vi "main 3rd.vi"() -> ()   [LabVIEW 2013]
uses:
  <vilib>/Utility/file.llb/Read From Spreadsheet File (DBL).vi
panel:
  out "数值 2":i32
  out "数值":i32
  out "From OD fit?":bool
  out "Current file num":i32
  out "ROI Width":u32
  out "ROI Height":u32
  in  "Image Dark":dbl[][](array[numeric])
  in  "Image Light":dbl[][](array[numeric])
  in  "Image Atom":dbl[][](array[numeric])
  out "Best fit parameters":dbl[](array[numeric])
  out "Fitting Results Save Path":string[](array[string])
  out "Best fit results":dbl[][](array[numeric])
  in  "Initial guess values":dbl[](array[numeric])
  in  "Latest image data":dbl[][](array[numeric])
  out "Fitting Type":u16(ring)
  out "Force Guess?":bool
  out "Aquired?":bool
  out "Process Index":i32
  out "External Trigger":bool
  out "XY图":cluster{dbl[], dbl[]}[](graph)
  out "OD Image":dbl[][](graph)
  in  "OD fit":bool
  in  "OD num":i32
  out "Fit Done":bool
  in  "Exit":bool
  out "XY图 2":cluster{dbl[], dbl[]}[](graph)
  in  "Auto Split":bool
  in  "Fit":bool
  in  "Open File":bool
  in  "Auto Fit":bool
  in  "Stop":bool
  in  "Aquire":bool
  in  "Fitting Config":bool
  in  "Camera Config":bool
  in  "Initialize":bool
  in  "Live Image Display":refnum<k7>(container)
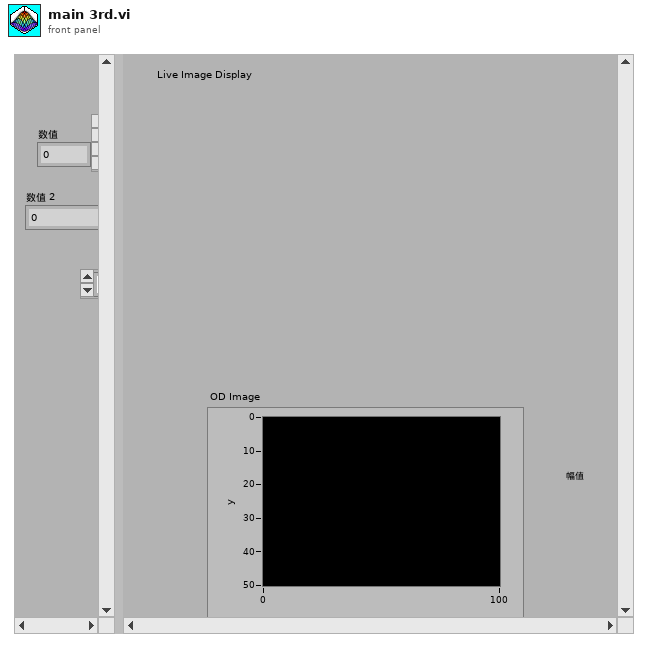
[diagram p1: front panel]
types:
  T1 = enum8{"Enabled", "Disabled", "Disabled and Grayed Out"}
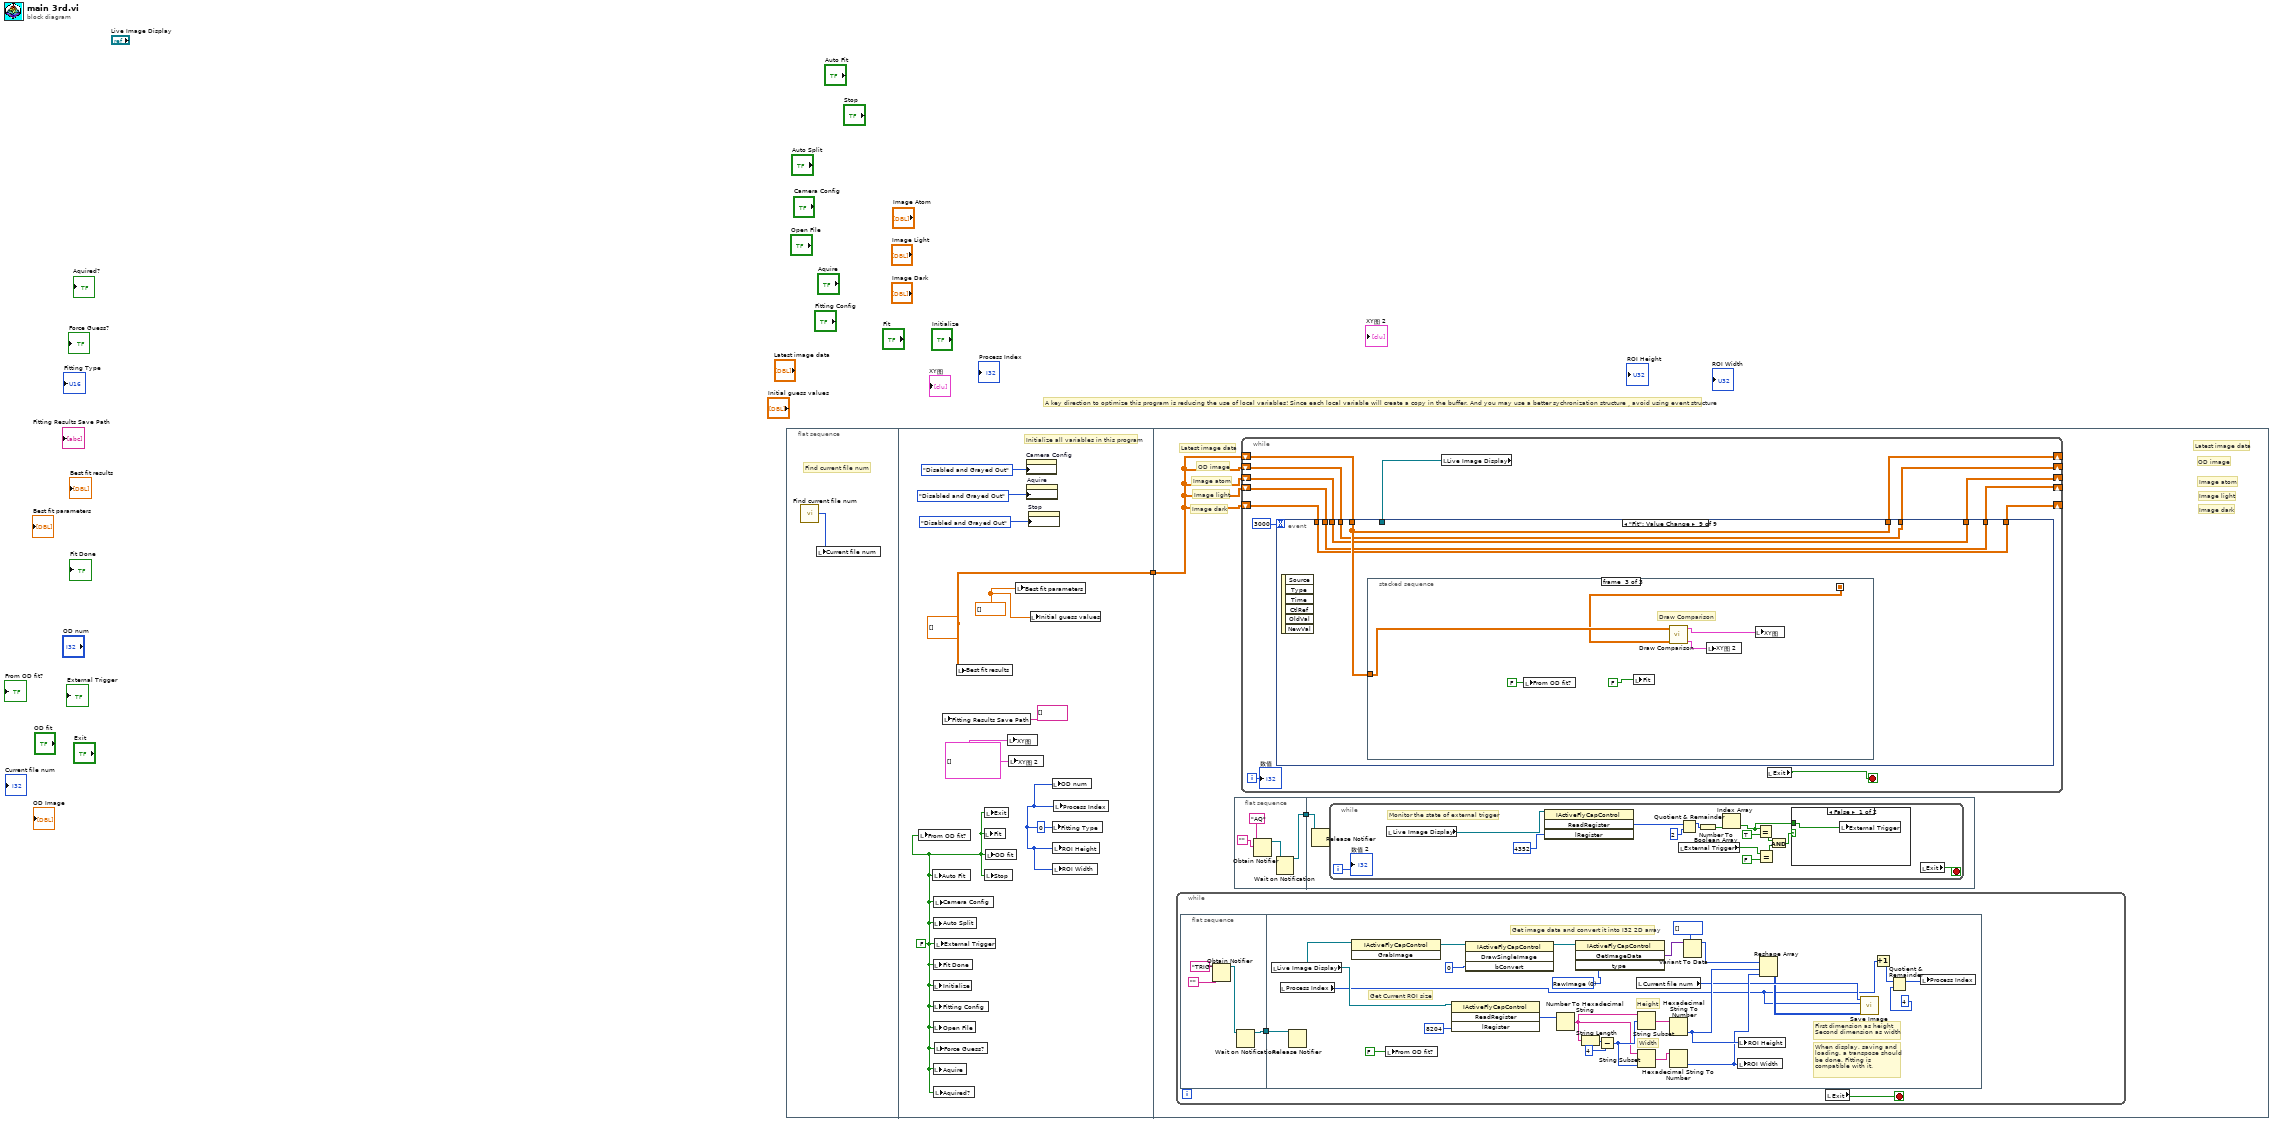
[diagram p0: block diagram]
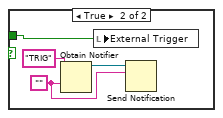
[diagram p2: hidden frame]
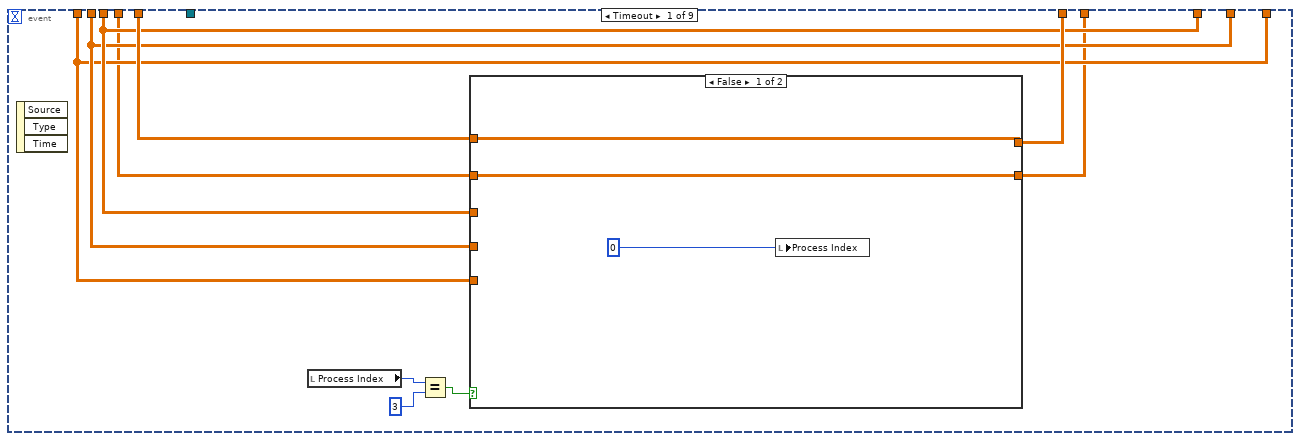
[diagram p3: hidden frame]
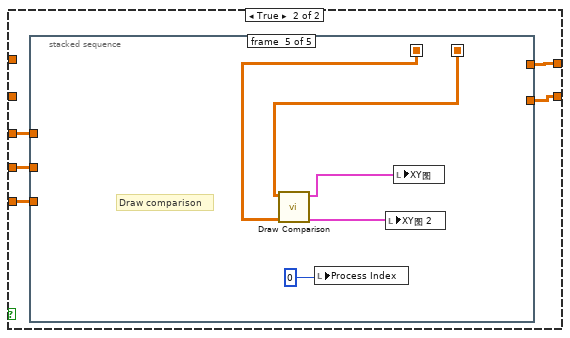
[diagram p4: hidden frame]
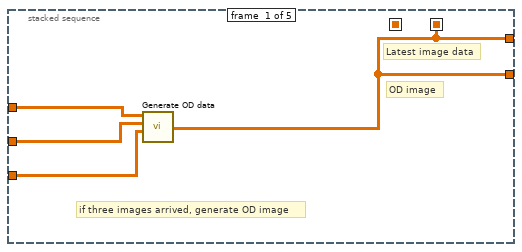
[diagram p5: hidden frame]
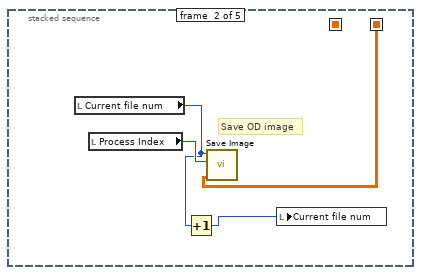
[diagram p6: hidden frame]
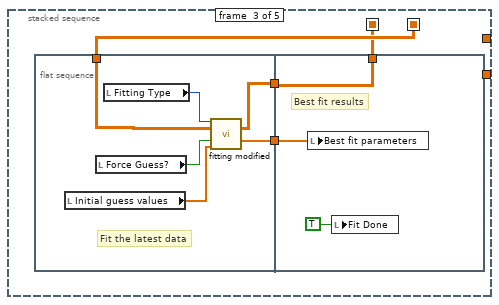
[diagram p7: hidden frame]
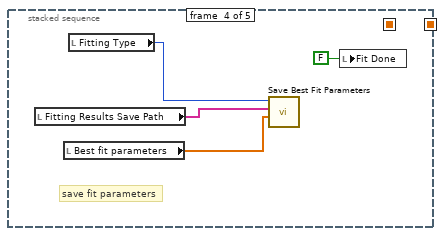
[diagram p8: hidden frame]
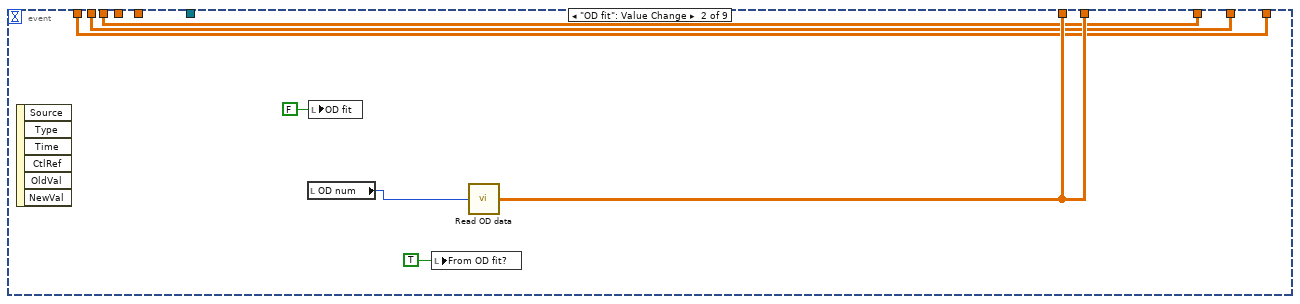
[diagram p9: hidden frame]
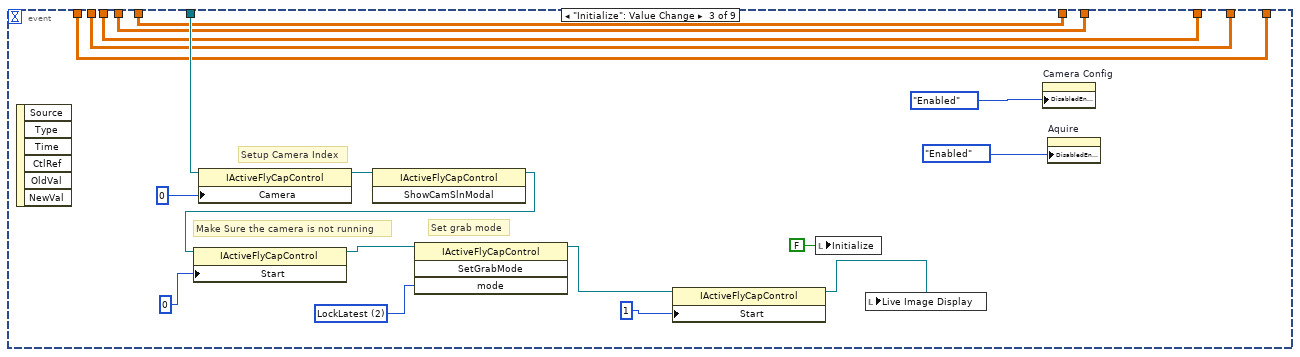
[diagram p10: hidden frame]
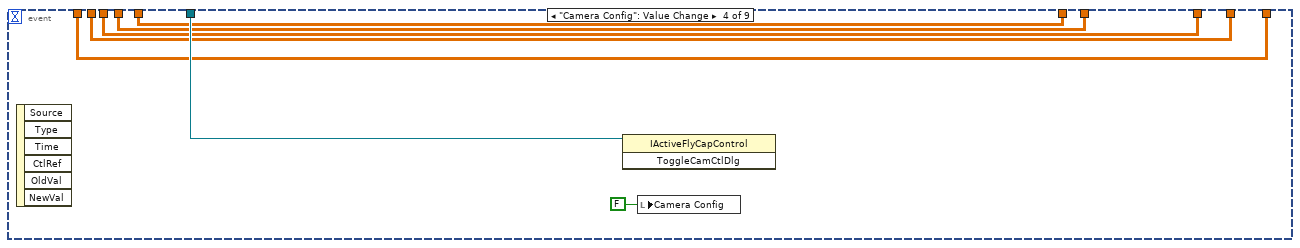
[diagram p11: hidden frame]
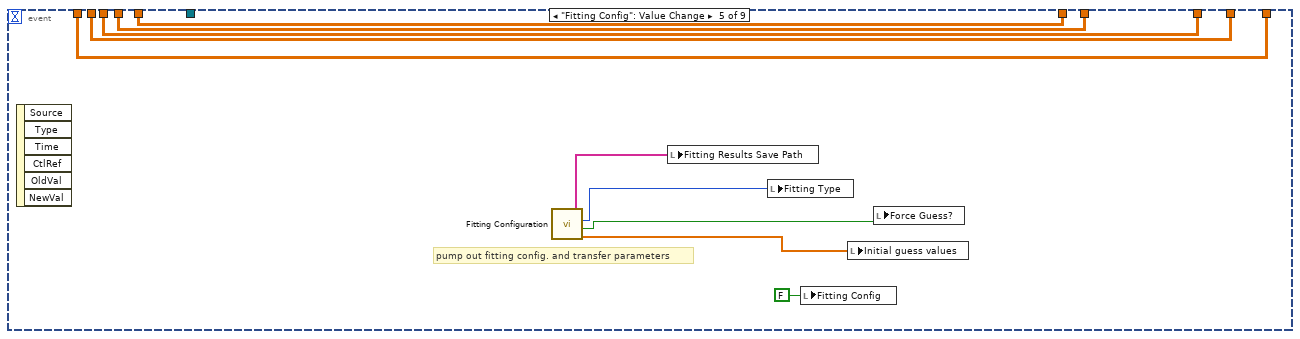
[diagram p12: hidden frame]
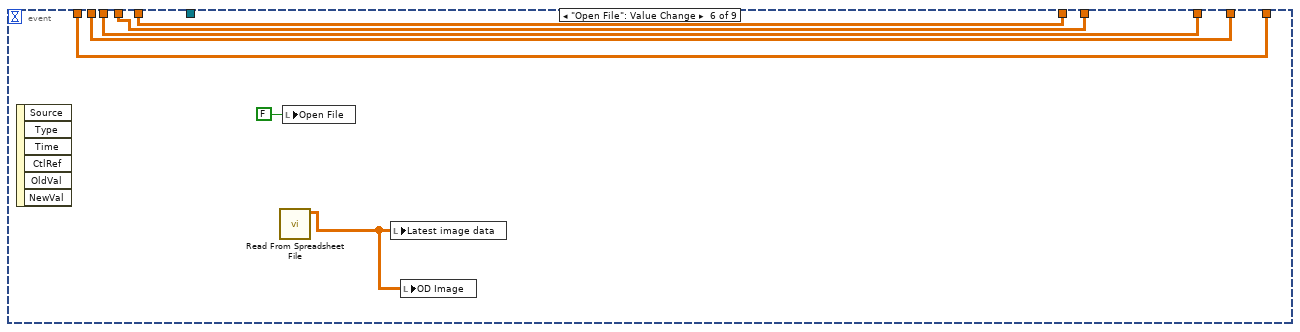
[diagram p13: hidden frame]
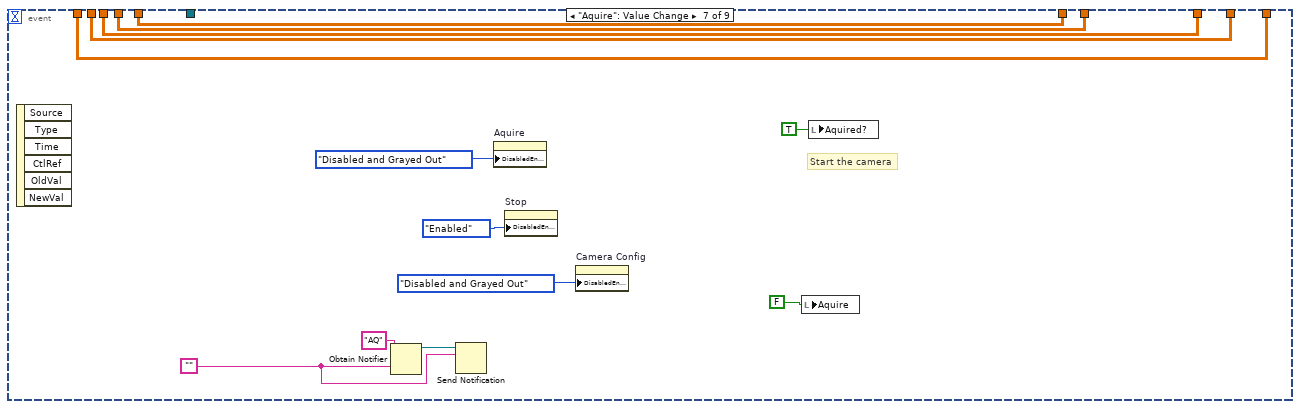
[diagram p14: hidden frame]
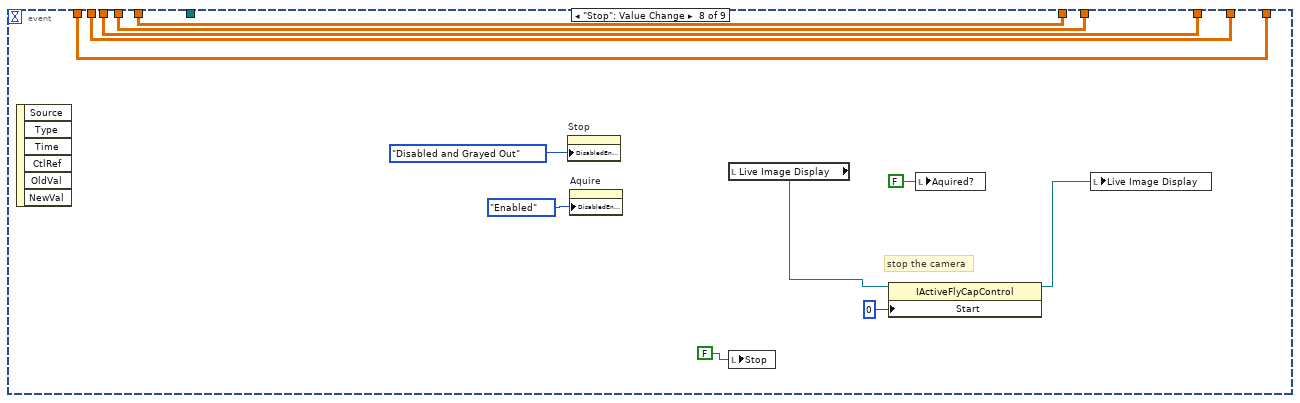
[diagram p15: hidden frame]
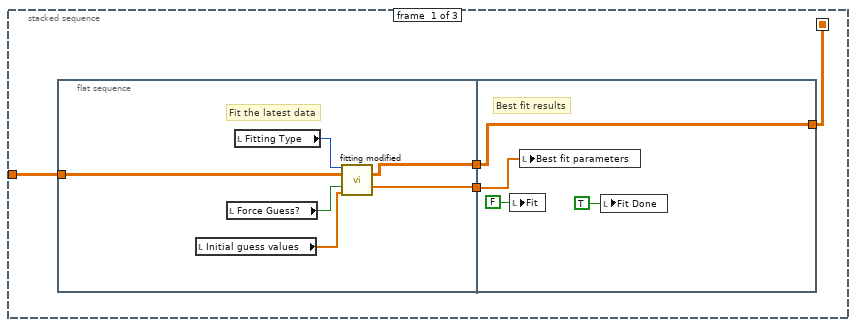
[diagram p16: hidden frame]
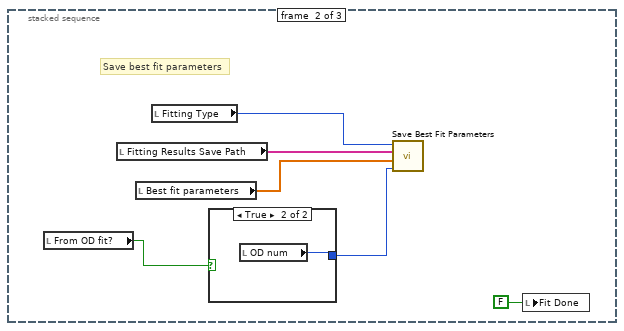
[diagram p17: hidden frame]
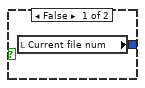
[diagram p18: hidden frame]
diagram:
  # "A key direction to optimize this program is reducing the use of local variables! Since each local variable will create a copy in the buffer. And you may use a better sychronization structure，avoid using event structure"
  n1 = flat-sequence {
    tunnel: [w5] -> w1
    tunnel: w1 -> [w13]
    frame #0 {
      # "Find current file num"
      n2 = call "Find current file num.vi"() -> ("Current File Num"=w2:u16)  [unwired: 2 in]
      n3 = local write "Current file num"(w2) -> ()
    }
    frame #1 {
      w7 = cluster{dbl[], dbl[]}[] [] ("XY图")
      w6 = 0 ("OD num")
      w5 = dbl[][] [] ("Best fit results")
      w4 = dbl[] [] ("Best fit parameters")
      w3 = FALSE ("Aquire")
      # "Initialize all variables in this program"
      n4 = local write "From OD fit?"(w3) -> ()
      n5 = local write "Auto Fit"(w3) -> ()
      n6 = local write "Auto Split"(w3) -> ()
      n7 = local write "Fit Done"(w3) -> ()
      n8 = local write "Initialize"(w3) -> ()
      n9 = local write "Fitting Config"(w3) -> ()
      n10 = local write "Open File"(w3) -> ()
      n11 = local write "Aquire"(w3) -> ()
      n12 = local write "Camera Config"(w3) -> ()
      n13 = local write "Aquired?"(w3) -> ()
      n14 = local write "Force Guess?"(w3) -> ()
      n15 = local write "External Trigger"(w3) -> ()
      n16 = local write "Fitting Results Save Path"(string[] [] ("Fitting Results Save Path")) -> ()
      n17 = local write "Best fit results"(w5) -> ()
      n18 = local write "Fit"(w3) -> ()
      n19 = local write "Exit"(w3) -> ()
      n20 = local write "Stop"(w3) -> ()
      n21 = local write "OD fit"(w3) -> ()
      n22 = local write "XY图"(w7) -> ()
      n23 = local write "XY图 2"(w7) -> ()
      n24 = local write "Best fit parameters"(w4) -> ()
      n25 = property on="Camera Config" class="Bool (strict)"("DisabledEnum"=T1."Disabled and Grayed Out" ("禁用")) -> ()  [unwired: 2 in, 2 out]
      n26 = property on="Aquire" class="Bool (strict)"("DisabledEnum"=T1."Disabled and Grayed Out" ("禁用")) -> ()  [unwired: 2 in, 2 out]
      n27 = property on="Stop" class="Bool (strict)"("DisabledEnum"=T1."Disabled and Grayed Out" ("禁用")) -> ()  [unwired: 2 in, 2 out]
      n28 = local write "Initial guess values"(w4) -> ()
      n29 = local write "OD num"(w6) -> ()
      n30 = local write "Fitting Type"(w6) -> ()
      n31 = local write "ROI Height"(w6) -> ()
      n32 = local write "ROI Width"(w6) -> ()
      n33 = local write "Process Index"(w6) -> ()
    }
    frame #2 {
      # "Image dark"
      # "Image light"
      # "Image atom"
      # "Image dark"
      # "Image light"
      # "Image atom"
      # "OD image"
      # "Latest image data"
      # "OD image"
      # "Latest image data"
      n34 = while {
        stop <- w40 stop-if-true
        n35 = flat-sequence {
          tunnel: [w41] -> w39
          tunnel: w39 -> [w53]
          frame #0 {
            n36 = Obtain Notifier(name (unnamed)="TRIG" ("名称（未命名）"), notification data type="") -> (notifier out=w42:refnum<notifier>)  [unwired: 2 in, 2 out]
            n37 = Wait on Notification(notifier=w42) -> (notifier out=w41:refnum<notifier>)  [unwired: 3 in, 3 out]
          }
          frame #1 {
            w70 = 0 items=["RawImage", "ColorProcessedImage"] ("type")
            # "Get image data and convert it into I32 2D array"
            # "When display, saving and \nloading, a transpose should\nbe done. Fitting is \ncompatible with it."
            # "First dimension as height\nSecond dimension as width"
            # "Width"
            # "Height"
            # "Get Current ROI size"
            n38 = local read "Live Image Display"() -> (w55:refnum<k7>)
            n39 = local read "Process Index"() -> (w48:i32)
            n40 = Release Notifier(notifier=w53) -> ()  [unwired: 2 in, 3 out]
            n41 = invoke class="IActiveFlyCapControl" method="GrabImage"(reference=w55) -> (reference out=w46:refnum<k7>)  [unwired: 2 in, 2 out]
            n42 = local write "From OD fit?"(FALSE ("From OD fit?")) -> ()
            n43 = invoke class="IActiveFlyCapControl" method="ReadRegister"(reference=w55, "lRegister"=u32 8204) -> ("ReadRegister"=w67:u32)  [unwired: 2 in, 3 out]
            n44 = invoke class="IActiveFlyCapControl" method="DrawSingleImage"(reference=w46, "bConvert"=0) -> (reference out=w47:refnum<k7>)  [unwired: 2 in, 3 out]
            n45 = Number To Hexadecimal String(2:w67) -> (0:w63:string)  [unwired: 1 in]
            n46 = invoke class="IActiveFlyCapControl" method="GetImageData"(reference=w47, "type"=w70) -> ("GetImageData"=w68:variant)  [unwired: 2 in, 3 out]
            n47 = String Length(string=w63) -> (length=w66:i32)
            n48 = Subtract(x=w66, y=4) -> (x-y=w64:i32)
            n49 = local read "Current file num"() -> (w54:i32)
            n50 = String Subset(string=w63, length (rest)=w64) -> (substring=w60:string)  [unwired: 1 in]
            n51 = String Subset(string=w63, offset (0)=w64) -> (substring=w61:string)  [unwired: 1 in]
            n52 = Hexadecimal String To Number(string=w60) -> (number=w57:u32)  [unwired: 2 in, 1 out]
            n53 = Hexadecimal String To Number(string=w61) -> (number=w58:u32)  [unwired: 2 in, 1 out]
            n54 = Variant To Data(type=i32[] [], Variant=w68) -> (data=w59:i32[])  [unwired: 1 in, 1 out]
            n55 = local write "ROI Width"(w57) -> ()
            n56 = local write "ROI Height"(w58) -> ()
            n57 = Reshape Array(w59, w58, w57) -> (w49:i32[][])
            n58 = call "Save Image.vi"("Data"=w49, "Process Index"=w48, "Current File Num"=w54) -> ()  [unwired: 9 in]
            n59 = Increment(x=w48) -> (x+1=w50:i32)
            n60 = Quotient & Remainder(x=w50, y=4) -> (x-y*floor(x/y)=w52:i32)  [unwired: 1 out]
            n61 = local write "Process Index"(w52) -> ()
          }
        }
        n62 = local read "Exit"() -> (w40:bool)
      }
      n63 = flat-sequence {
        tunnel: [w14] -> w12
        tunnel: w12 -> [w18]
        frame #0 {
          n64 = Obtain Notifier(name (unnamed)="AQ" ("名称（未命名）"), notification data type="") -> (notifier out=w16:refnum<notifier>)  [unwired: 2 in, 2 out]
          n65 = Wait on Notification(notifier=w16) -> (notifier out=w14:refnum<notifier>)  [unwired: 3 in, 3 out]
        }
        frame #1 {
          n66 = Release Notifier(notifier=w18) -> ()  [unwired: 2 in, 3 out]
          n67 = while {
            i -> [w32]
            stop <- w33 stop-if-true
            # "Monitor the state of external trigger"
            n68 = local read "Live Image Display"() -> (w31:refnum<k7>)
            n69 = invoke class="IActiveFlyCapControl" method="ReadRegister"(reference=w31, "lRegister"=u32 4352) -> ("ReadRegister"=w29:u32)  [unwired: 2 in, 3 out]
            n70 = local read "External Trigger"() -> (w24:bool)
            n71 = Quotient & Remainder(x=w29, y=u32 2) -> (x-y*floor(x/y)=w27:u32)  [unwired: 1 out]
            n72 = Number To Boolean Array(number=w27) -> (Boolean array=w26:bool[])
            n73 = Index Array(array=w26) -> (element=w19:bool)  [unwired: 1 in]
            n74 = Equal?(x=w19, y=TRUE) -> (x = y?=w21:bool)
            n75 = Equal?(x=w24, y=FALSE) -> (x = y?=w22:bool)
            n76 = And(x=w21, y=w22) -> (x .and. y?=w20:bool)
            n77 = case shown="False" w20 {
              tunnel: w19 -> [w34 w38]
              frame False {
                n78 = local write "External Trigger"(w34) -> ()
              }
              frame True {
                w35 = ""
                n79 = Obtain Notifier(name (unnamed)="TRIG" ("名称（未命名）"), notification data type=w35) -> (notifier out=w36:refnum<notifier>)  [unwired: 2 in, 2 out]
                n80 = local write "External Trigger"(w38) -> ()
                n81 = Send Notification(notification=w35, notifier=w36) -> ()  [unwired: 1 in, 2 out]
              }
            }
            n82 = local read "Exit"() -> (w33:bool)
            "数值 2" <- w32
          }
        }
      }
      n83 = while {
        shift-right: [w82] -> _
        shift-left: w13 -> [w81]
        shift-right: [w76] -> _
        shift-left: w13 -> [w73]
        shift-right: [w75] -> _
        shift-left: w13 -> [w79]
        shift-right: [w74] -> _
        shift-left: w13 -> [w78]
        shift-right: [w80] -> _
        shift-left: w13 -> [w77]
        i -> [w72]
        stop <- w83 stop-if-true
        n84 = local read "Live Image Display"() -> (w84:refnum<k7>)
        n85 = event shown="[8] \"Fit\": Value Change" {
          selector: _ -> [_ _ _ _ _ _ _ _ _]
          dyn-events: _ -> [_ _ _ _ _ _ _ _ _]
          timeout: 3000 -> [_ _ _ _ _ _ _ _ _]
          tunnel: w84 -> [_ _ w151 w164 _ _ _ _ _]
          tunnel: [w91 w137 w147 w162 w169 w179 w189 w199 w211] -> w82
          tunnel: w81 -> [w90 _ w147 w162 w169 w179 w189 w199 w211]
          tunnel: w73 -> [w86 _ w146 w161 w168 w178 w188 w198 w210]
          tunnel: [w87 w134 w143 w158 w165 w175 w185 w195 w207] -> w80
          tunnel: w79 -> [w89 w136 w145 w160 w167 w177 w187 w197 w209]
          tunnel: w78 -> [w88 w135 w144 w159 w166 w176 w186 w196 w208]
          tunnel: w77 -> [w87 w134 w143 w158 w165 w175 w185 w195 w207]
          tunnel: [w85 w137 w146 w161 w168 w178 w188 w198 w210] -> w76
          tunnel: [w89 w136 w145 w160 w167 w177 w187 w197 w209] -> w75
          tunnel: [w88 w135 w144 w159 w166 w176 w186 w196 w208] -> w74
          event Timeout {
            n86 = event-data() -> ()  [unwired: 1 in, 3 out]
            n87 = local read "Process Index"() -> (w94:i32)
            n88 = Equal?(x=w94, y=3) -> (x = y?=w92:bool)
            n89 = case shown="False" w92 {
              tunnel: w89 -> [_ w102]
              tunnel: w88 -> [_ w101]
              tunnel: w87 -> [_ w100]
              tunnel: [w96 w99] -> w91
              tunnel: w90 -> [w96 _]
              tunnel: w86 -> [w95 _]
              tunnel: [w95 w98] -> w85
              frame False {
                n90 = local write "Process Index"(0 ("Process Index")) -> ()
              }
              frame True {
                n91 = stacked-sequence {
                  seq-local: [w103 _ _ _ _] -> [_ w109 w112 _ w129]
                  seq-local: [_ _ w111 _ _] -> [_ _ _ _ w128]
                  tunnel: w102 -> [w106 _ _ _ _]
                  tunnel: w101 -> [w105 _ _ _ _]
                  tunnel: w100 -> [w104 _ _ _ _]
                  tunnel: [w103 _ _ _ _] -> w99
                  tunnel: [w103 _ _ _ _] -> w98
                  frame #0 {
                    # "OD image"
                    # "Latest image data"
                    # "if three images arrived, generate OD image"
                    n92 = call "Generate OD data.vi"("dark"=w104, "light"=w105, "atom"=w106) -> ("OD image"=w103:dbl[][])  [unwired: 3 in]
                  }
                  frame #1 {
                    # "Save OD image"
                    n93 = local read "Current file num"() -> (w108:i32)
                    n94 = local read "Process Index"() -> (w110:i32)
                    n95 = Increment(x=w108) -> (x+1=w107:i32)
                    n96 = call "Save Image.vi"("Data"=w109, "Process Index"=w110, "Current File Num"=w108) -> ()  [unwired: 9 in]
                    n97 = local write "Current file num"(w107) -> ()
                  }
                  frame #2 {
                    n98 = flat-sequence {
                      tunnel: [w117] -> w114
                      tunnel: [w116] -> w113
                      tunnel: w112 -> [w115]
                      tunnel: w114 -> [w121]
                      tunnel: w113 -> [w123]
                      tunnel: [w121] -> w111
                      frame #0 {
                        # "Fit the latest data"
                        n99 = local read "Initial guess values"() -> (w118:dbl[])
                        n100 = local read "Force Guess?"() -> (w119:bool)
                        n101 = local read "Fitting Type"() -> (w120:u16)
                        n102 = call "fitting modified.vi"("fitting type"=w120, "2D data"=w115, "force guess?"=w119, "intial guess value"=w118) -> ("best fit"=w117:dbl[][], "best fit parameters"=w116:dbl[])  [unwired: 9 in, 1 out]
                      }
                      frame #1 {
                        # "Best fit results"
                        n103 = local write "Best fit parameters"(w123) -> ()
                        n104 = local write "Fit Done"(TRUE ("Fit Done")) -> ()
                      }
                    }
                  }
                  frame #3 {
                    # "save fit parameters"
                    n105 = local read "Fitting Results Save Path"() -> (w126:string[])
                    n106 = local read "Best fit parameters"() -> (w125:dbl[])
                    n107 = local read "Fitting Type"() -> (w127:u16)
                    n108 = call "Save Best Fit Parameters.vi"("Best Fit Parameters"=w125, "Fitting Results Save Path"=w126, "Fitting Type"=w127) -> ()  [unwired: 9 in]
                    n109 = local write "Fit Done"(FALSE ("Fit Done")) -> ()
                  }
                  frame #4 {
                    # "Draw comparison"
                    n110 = call "Draw Comparison.vi"("Best Fit"=w128, "Raw Data"=w129) -> ("Vertical Comparison"=w131:cluster{i32[], dbl[]}[], "Horizontal Comparison"=w132:cluster{i32[], dbl[]}[])  [unwired: 7 in]
                    n111 = local write "Process Index"(0 ("Process Index")) -> ()
                    n112 = local write "XY图 2"(w131) -> ()
                    n113 = local write "XY图"(w132) -> ()
                  }
                }
              }
            }
          }
          event "OD fit": Value Change {
            n114 = event-data() -> ()  [unwired: 1 in, 6 out]
            n115 = local read "OD num"() -> (w138:i32)
            n116 = local write "OD fit"(FALSE ("OD fit")) -> ()
            n117 = local write "From OD fit?"(TRUE ("From OD fit?")) -> ()
            n118 = call "Read OD data.vi"("OD num"=w138) -> ("OD data"=w137:dbl[][])  [unwired: 4 in]
          }
          event "Initialize": Value Change {
            w155 = 2 items=["FreeRunning", "LockNext", "LockLatest"] ("mode")
            # "Setup Camera Index"
            # "Set grab mode"
            # "Make Sure the camera is not running"
            n119 = event-data() -> ()  [unwired: 1 in, 6 out]
            n120 = property class="IActiveFlyCapControl"(reference=w151, "Camera"=0 ("Start")) -> (reference out=w154:refnum<k7>)  [unwired: 1 in, 1 out]
            n121 = invoke class="IActiveFlyCapControl" method="ShowCamSlnModal"(reference=w154) -> (reference out=w150:refnum<k7>)  [unwired: 2 in, 2 out]
            n122 = property class="IActiveFlyCapControl"(reference=w150, "Start"=0 ("Camera")) -> (reference out=w149:refnum<k7>)  [unwired: 1 in, 1 out]
            n123 = invoke class="IActiveFlyCapControl" method="SetGrabMode"(reference=w149, "mode"=w155) -> (reference out=w141:refnum<k7>)  [unwired: 2 in, 3 out]
            n124 = property class="IActiveFlyCapControl"(reference=w141, "Start"=1) -> (reference out=w140:refnum<k7>)  [unwired: 1 in, 1 out]
            n125 = local write "Initialize"(FALSE ("Initialize")) -> ()
            n126 = local write "Live Image Display"(w140) -> ()
            n127 = property on="Camera Config" class="Bool (strict)"("DisabledEnum"=T1."Enabled" ("禁用")) -> ()  [unwired: 2 in, 2 out]
            n128 = property on="Aquire" class="Bool (strict)"("DisabledEnum"=T1."Enabled" ("禁用")) -> ()  [unwired: 2 in, 2 out]
          }
          event "Camera Config": Value Change {
            n129 = event-data() -> ()  [unwired: 1 in, 6 out]
            n130 = invoke class="IActiveFlyCapControl" method="ToggleCamCtlDlg"(reference=w164) -> ()  [unwired: 2 in, 3 out]
            n131 = local write "Camera Config"(FALSE ("Camera Config")) -> ()
          }
          event "Fitting Config": Value Change {
            # "pump out fitting config. and transfer parameters"
            n132 = event-data() -> ()  [unwired: 1 in, 6 out]
            n133 = call "Fitting Configuration.vi"() -> ("intial guess"=w170:dbl[], "Force Guess？"=w171:bool, "Fitting Type"=w173:u16, "Fitting Results Save Path"=w172:string[])  [unwired: 5 in]
            n134 = local write "Fitting Results Save Path"(w172) -> ()
            n135 = local write "Fitting Type"(w173) -> ()
            n136 = local write "Fitting Config"(FALSE ("Fitting Config")) -> ()
            n137 = local write "Initial guess values"(w170) -> ()
            n138 = local write "Force Guess?"(w171) -> ()
          }
          event "Open File": Value Change {
            n139 = event-data() -> ()  [unwired: 1 in, 6 out]
            n140 = call-poly <vilib>:"Read From Spreadsheet File.vi"() -> ("all rows"=w180:dbl[][])  [unwired: 7 in, 4 out]
            n141 = local write "Open File"(FALSE ("Open File")) -> ()
            n142 = local write "Latest image data"(w180) -> ()
            n143 = local write "OD Image"(w180) -> ()
          }
          event "Aquire": Value Change {
            w182 = ""
            # "Start the camera"
            n144 = event-data() -> ()  [unwired: 1 in, 6 out]
            n145 = Obtain Notifier(name (unnamed)="AQ" ("名称（未命名）"), notification data type=w182) -> (notifier out=w183:refnum<notifier>)  [unwired: 2 in, 2 out]
            n146 = Send Notification(notification=w182, notifier=w183) -> ()  [unwired: 1 in, 2 out]
            n147 = property on="Aquire" class="Bool (strict)"("DisabledEnum"=T1."Disabled and Grayed Out" ("禁用")) -> ()  [unwired: 2 in, 2 out]
            n148 = property on="Stop" class="Bool (strict)"("DisabledEnum"=T1."Enabled" ("禁用")) -> ()  [unwired: 2 in, 2 out]
            n149 = property on="Camera Config" class="Bool (strict)"("DisabledEnum"=T1."Disabled and Grayed Out" ("禁用")) -> ()  [unwired: 2 in, 2 out]
            n150 = local write "Aquire"(FALSE ("Initialize")) -> ()
            n151 = local write "Aquired?"(TRUE ("Aquired?")) -> ()
          }
          event "Stop": Value Change {
            # "stop the camera"
            n152 = event-data() -> ()  [unwired: 1 in, 6 out]
            n153 = property on="Stop" class="Bool (strict)"("DisabledEnum"=T1."Disabled and Grayed Out" ("禁用")) -> ()  [unwired: 2 in, 2 out]
            n154 = property on="Aquire" class="Bool (strict)"("DisabledEnum"=T1."Enabled" ("禁用")) -> ()  [unwired: 2 in, 2 out]
            n155 = local read "Live Image Display"() -> (w202:refnum<k7>)
            n156 = local write "Stop"(FALSE ("Initialize")) -> ()
            n157 = property class="IActiveFlyCapControl"(reference=w202, "Start"=0) -> (reference out=w201:refnum<k7>)  [unwired: 1 in, 1 out]
            n158 = local write "Aquired?"(FALSE ("Aquired?")) -> ()
            n159 = local write "Live Image Display"(w201) -> ()
          }
          event "Fit": Value Change {
            n160 = event-data() -> ()  [unwired: 1 in, 6 out]
            n161 = stacked-sequence {
              seq-local: [w212 _ _] -> [_ _ w235]
              tunnel: w211 -> [w213 _ w236]
              frame #0 {
                n162 = flat-sequence {
                  tunnel: [w218] -> w215
                  tunnel: [w217] -> w214
                  tunnel: w213 -> [w216]
                  tunnel: w215 -> [w222]
                  tunnel: w214 -> [w225]
                  tunnel: [w222] -> w212
                  frame #0 {
                    # "Fit the latest data"
                    n163 = local read "Initial guess values"() -> (w220:dbl[])
                    n164 = local read "Force Guess?"() -> (w221:bool)
                    n165 = local read "Fitting Type"() -> (w219:u16)
                    n166 = call "fitting modified.vi"("fitting type"=w219, "2D data"=w216, "force guess?"=w221, "intial guess value"=w220) -> ("best fit"=w218:dbl[][], "best fit parameters"=w217:dbl[])  [unwired: 9 in, 1 out]
                  }
                  frame #1 {
                    # "Best fit results"
                    n167 = local write "Fit"(FALSE ("Fit")) -> ()
                    n168 = local write "Best fit parameters"(w225) -> ()
                    n169 = local write "Fit Done"(TRUE ("Fit Done")) -> ()
                  }
                }
              }
              frame #1 {
                # "Save best fit parameters"
                n170 = local read "From OD fit?"() -> (w227:bool)
                n171 = local read "Fitting Results Save Path"() -> (w229:string[])
                n172 = local read "Best fit parameters"() -> (w228:dbl[])
                n173 = local read "Fitting Type"() -> (w230:u16)
                n174 = case shown="True" w227 {
                  tunnel: [w232 w233] -> w226
                  frame False {
                    n175 = local read "Current file num"() -> (w232:i32)
                  }
                  frame True {
                    n176 = local read "OD num"() -> (w233:i32)
                  }
                }
                n177 = call "Save Best Fit Parameters.vi"("Current File Num"=w226, "Best Fit Parameters"=w228, "Fitting Results Save Path"=w229, "Fitting Type"=w230) -> ()  [unwired: 8 in]
                n178 = local write "Fit Done"(FALSE ("Fit Done")) -> ()
              }
              frame #2 {
                # "Draw Comparison"
                n179 = local write "From OD fit?"(FALSE ("From OD fit?")) -> ()
                n180 = local write "Fit"(FALSE ("Initialize")) -> ()
                n181 = call "Draw Comparison.vi"("Best Fit"=w235, "Raw Data"=w236) -> ("Vertical Comparison"=w238:cluster{i32[], dbl[]}[], "Horizontal Comparison"=w239:cluster{i32[], dbl[]}[])  [unwired: 7 in]
                n182 = local write "XY图 2"(w238) -> ()
                n183 = local write "XY图"(w239) -> ()
              }
            }
          }
        }
        n184 = local read "Exit"() -> (w83:bool)
        "数值" <- w72
      }
    }
  }
